vi "Info by Node ID.vi"(8 "error in (no error)":errorcluster, 10 "Node ID":u32, 11 "TCPMessageAPI in":refnum<class "TCPMessageAPI.lvclass">) -> (0 "error out":errorcluster, 2 "Client Info":T1, 3 "TCPMessageAPI out":refnum<class "TCPMessageAPI.lvclass">)   [LabVIEW 2020]
uses:
  TCPMessageAPI.lvclass/TCPMessageAPI.ctl
  TCPMessageAPI.lvclass
  C:/dev/lv 2020/lv-vecto/Vecto/TCPMessageService/TCPMessageAPI.lvclass
  C:/Program Files (x86)/National Instruments/LabVIEW 2024/vi.lib/IlluminatedG/IG HTTP Server/HTTP Server/Service/Service.lvclass
  proto/TcpClientHello/Data.ctl
  proto/TcpClientHello/TcpClientHello.lvlib
  Client Info.ctl
  Vecto.lvlib
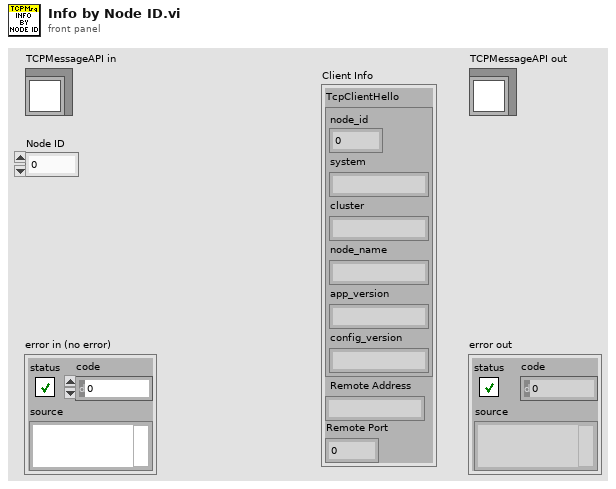
[diagram p1: front panel]
types:
  T1 = typedef "Vecto.lvlib/Client Info.ctl" = cluster{"TcpClientHello":T2, "Remote Address":string, "Remote Port":u16}
  T2 = typedef "TcpClientHello.lvlib/Data.ctl" = cluster{"node_id":u32, "system":string, "cluster":string, "node_name":string, "app_version":string, "config_version":string}
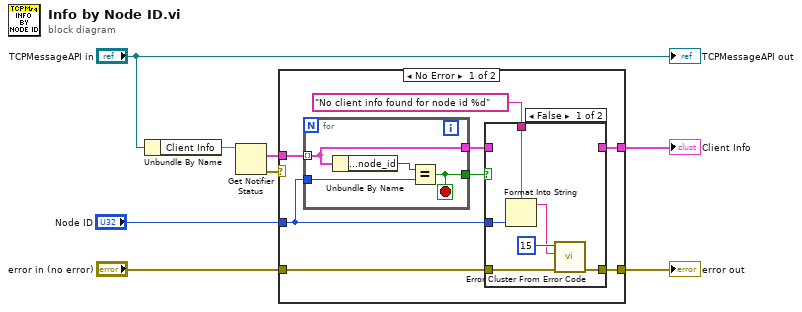
[diagram p0: block diagram]
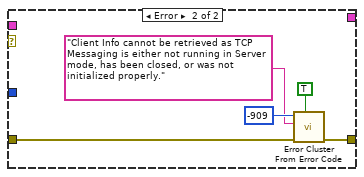
[diagram p3: hidden frame]
diagram:
  n1 = Unbundle By Name("TCPMessageAPI in") -> ("Client Info"=w7)
  n2 = Get Notifier Status(notifier=w7) -> (current notification=w2:T1[], error out=w1:errorcluster)  [unwired: 1 in, 3 out]
  n3 = case shown="No Error" w1 {
    tunnel: [w14 _] -> w6
    tunnel: "error in (no error)" -> [w13 w33]
    tunnel: [w12 w32] -> w4
    tunnel: "Node ID" -> [w11 _]
    tunnel: w2 -> [w9 _]
    frame No Error {
      n4 = for {
        tunnel: w9 -> [w25] mode=indexing
        tunnel: w11 -> [w28]
        tunnel: [w25] -> w15
        tunnel: [w26] -> w16
        stop <- w26 stop-if-true
        n5 = Unbundle By Name(w25) -> ("TcpClientHello.node_id"=w27:u32)
        n6 = Equal?(x=w27, y=w28) -> (x = y?=w26:bool)
      }
      n7 = case shown="False" w16 {
        tunnel: w15 -> [_ w24]
        tunnel: [_ w24] -> w14
        tunnel: w13 -> [w22 w23]
        tunnel: [w20 w23] -> w12
        tunnel: w11 -> [w19 _]
        tunnel: "No client info found for node id %d" -> [w18 _]
        frame False {
          n8 = Format Into String(format string=w18, w19) -> (resulting string=w17:string)  [unwired: 2 in, 1 out]
          n9 = call <vilib>:"Error Cluster From Error Code.vi"("error in (no error)"=w22, "error message (\"\")"=w17, "error code (0)"=15) -> ("error out"=w20:errorcluster)  [unwired: 6 in]
        }
        frame True {
        }
      }
    }
    frame Error {
      n10 = call <vilib>:"Error Cluster From Error Code.vi"("show call chain? (False)"=TRUE, "error in (no error)"=w33, "error message (\"\")"="Client Info cannot be retrieved as TCP Messaging is either not running in Server mode, has been closed, or was not initialized properly.", "error code (0)"=-909) -> ("error out"=w32:errorcluster)  [unwired: 5 in]
    }
  }
  "error out" <- w4
  "Client Info" <- w6
  "TCPMessageAPI out" <- "TCPMessageAPI in"
